vi "ScanEngine_SLM.vi"(7 "Action":T2, 8 "Metric Control":T3, 11 "Holo Array In":T1[](array[typedef]) {"Modes"."Amplititute" step=0.05}) -> (0 "Metric Image":sgl[][](array[numeric]), 2 "Metric Result":dbl)   [LabVIEW 2014]
uses:
  Controls/MetricControl_SLM.ctl
  Controls/Scan Metric_SLM.ctl
  Controls/ScanEngineState_SLM.ctl
  Controls/Holo Settings.ctl
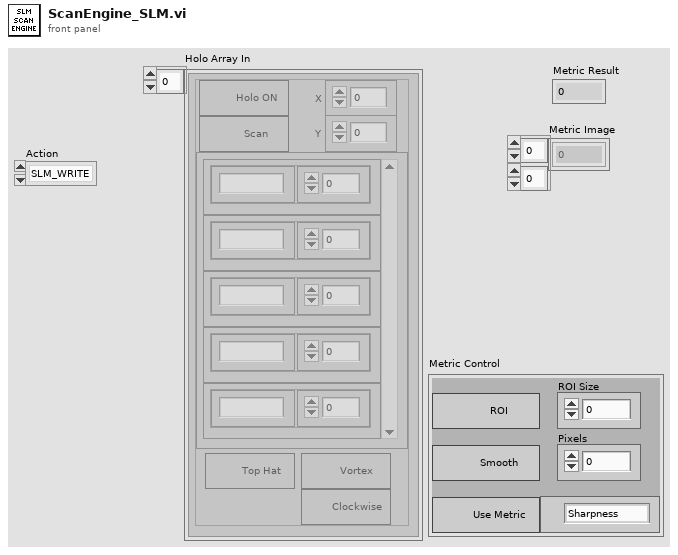
[diagram p1: front panel]
types:
  T1 = typedef "Holo Settings.ctl" = cluster{"Top Hat":bool, "Modes":cluster{"Mode ID":string, "Amplititute":dbl}[], "Vortex":bool, "Clockwise":bool, "X":dbl, "Y":dbl, "Holo ON":bool, "Scan":bool}
  T2 = typedef "ScanEngineState_SLM.ctl" = enum16{"SLM_WRITE", "IMAGE", ""}
  T3 = typedef "MetricControl_SLM.ctl" = cluster{"Use Metric":bool, "SLM Metric":T4, "Smooth":bool, "Pixels":dbl, "ROI":bool, "ROI Size":dbl}
  T4 = typedef "Scan Metric_SLM.ctl" = enum16{"Sharpness", "Brightness", "Combined"}
  T5 = typedef "Image Acquisition Parameters.ctl" = cluster{"Scan Type":enum16{"Sample Scanning", "Beam Scanning"}, "Scan Mode":enum16{"XY", "XZ", "YZ", "XYZ"}, "Fast Axis Frequency (Hz)":dbl, "Image Format":u16, "Line Accumulations":u16, "Frames Per Capture":u16, "Frames Accumulations":u16, "Image Dimension (um)":dbl[], "Number of Z Steps":u8, "Z Steps Size (um)":dbl, "Pixel Size (nm)":dbl[]}
  T6 = typedef "SLM General Settings.ctl" = cluster{"Holo size (pixels)":i32, "Top hat radius":dbl, "Number of modes":i32, "Bkg gradient X":dbl, "Bkg gradient Y":dbl, "Flat":bool, "Mode Matrix":u16}
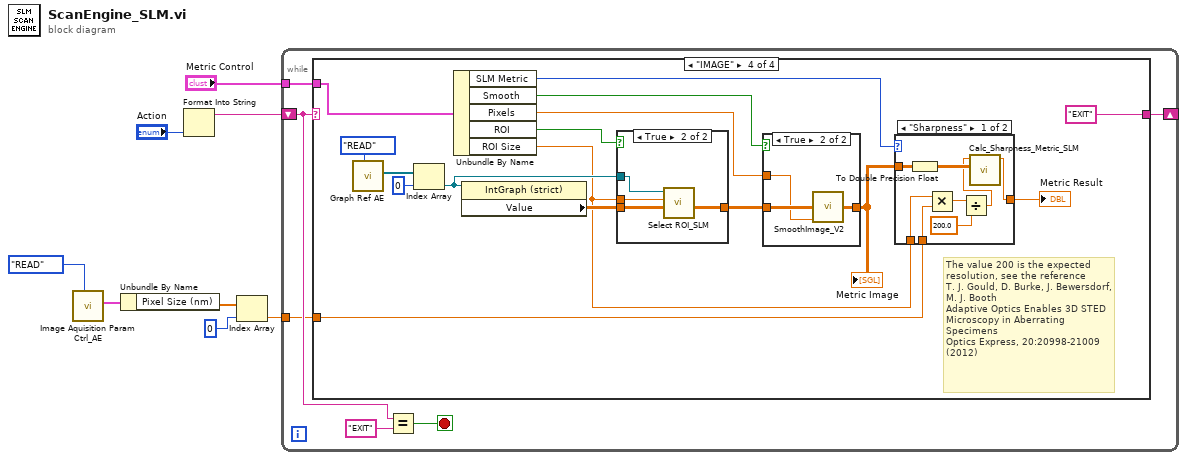
[diagram p0: block diagram]
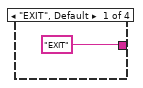
[diagram p2: hidden frame]
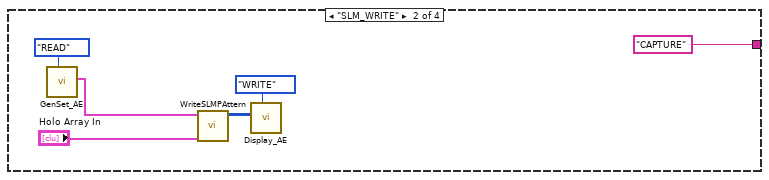
[diagram p3: hidden frame]
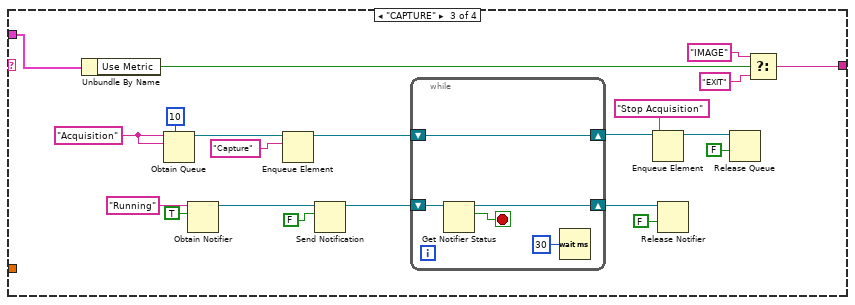
[diagram p4: hidden frame]
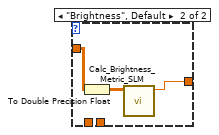
[diagram p6: hidden frame]
diagram:
  n1 = call "Image Aquisition Param Ctrl_AE.vi"("Action"=enum16{"READ", "WRITE"}."READ") -> ("Image Acquisition Parameters Out"=w4:T5)  [unwired: 10 in]
  n2 = Unbundle By Name(w4) -> ("Pixel Size (nm)"=w3:dbl[])
  n3 = Format Into String("Action") -> (resulting string=w6:string)  [unwired: 3 in, 1 out]
  n4 = Index Array(array=w3, index=0) -> (element=w1:dbl)
  n5 = while {
    shift-right: [w14] -> _
    shift-left: w6 -> [w13]
    tunnel: "Metric Control" -> [w10]
    tunnel: w1 -> [w9]
    stop <- w11 stop-if-true
    n6 = case shown="\"IMAGE\"" w13 {
      tunnel: ["EXIT" "CAPTURE" w39 "EXIT"] -> w14
      tunnel: w10 -> [_ _ w28 w60]
      tunnel: w9 -> [_ _ _ w48]
      frame "EXIT", Default {
      }
      frame "SLM_WRITE" {
        n7 = call "GenSet_AE.vi"("Enum"=enum16{"READ", "WRITE"}."READ") -> ("General settings Out"=w18:T6)  [unwired: 10 in]
        n8 = call "WriteSLMPAttern.vi"("Holo Array"="Holo Array In", "General settings"=w18) -> ("Display Array"=w17:u8[][])  [unwired: 9 in]
        n9 = call "Display_AE.vi"("Action"=enum16{"READ", "WRITE"}."WRITE", "Display Array In"=w17) -> ()  [unwired: 9 in, 1 out]
      }
      frame "CAPTURE" {
        w36 = "Acquisition" ("name (unnamed)")
        n10 = Unbundle By Name(w28) -> ("Use Metric"=w27:bool)
        n11 = Obtain Queue(max queue size (-1, unlimited)=10, name (unnamed)=w36, element data type=w36) -> (queue out=w34:refnum<queue>)  [unwired: 2 in, 2 out]
        n12 = Obtain Notifier(name (unnamed)="Running", notification data type=TRUE) -> (notifier out=w31:refnum<notifier>)  [unwired: 2 in, 2 out]
        n13 = Enqueue Element(queue=w34, element="Capture") -> (queue out=w24:refnum<queue>)  [unwired: 2 in, 2 out]
        n14 = Send Notification(notification=FALSE, notifier=w31) -> (notifier out=w40:refnum<notifier>)  [unwired: 1 in, 1 out]
        n15 = while {
          shift-right: [w43] -> w25
          shift-left: w24 -> [w43]
          shift-right: [w44] -> w30
          shift-left: w40 -> [w47]
          stop <- w46 stop-if-true
          n16 = Get Notifier Status(notifier=w47) -> (notifier out=w44:refnum<notifier>, current notification=w46:bool)  [unwired: 1 in, 3 out]
          n17 = Wait (ms)(milliseconds to wait=u32 30) -> ()  [unwired: 1 out]
        }
        n18 = Enqueue Element(queue=w25, element="Stop Acquisition") -> (queue out=w23:refnum<queue>)  [unwired: 2 in, 2 out]
        n19 = Release Notifier(notifier=w30, force destroy? (F)=FALSE) -> ()  [unwired: 1 in, 3 out]
        n20 = Release Queue(queue=w23, force destroy? (F)=FALSE) -> ()  [unwired: 1 in, 3 out]
        n21 = Select(t="IMAGE", s=w27, f="EXIT") -> (s? t:f=w39:string)
      }
      frame "IMAGE" {
        # "The value 200 is the expected\nresolution, see the reference\nT. J. Gould, D. Burke, J. Bewersdorf, M. J. Booth\nAdaptive Optics Enables 3D STED Microscopy in Aberrating Specimens\nOptics Express, 20:20998-21009 (2012)"
        n22 = call "Graph Ref AE.vi"("Action"=enum16{"READ", "WRITE"}."READ") -> ("Graph Ref Out"=w55:refnum<vi>[])  [unwired: 10 in]
        n23 = Index Array(array=w55, index=0) -> (element=w50:refnum<vi>)
        n24 = Unbundle By Name(w60) -> ("SLM Metric"=w59:T4, "Smooth"=w57:bool, "Pixels"=w58:dbl, "ROI"=w53:bool, "ROI Size"=w49:dbl)
        n25 = property class="IntGraph (strict)"(reference=w50) -> ("Value"=w51:sgl[][])  [unwired: 1 in, 2 out]
        n26 = case shown="True" w53 {
          tunnel: w51 -> [w64 w68]
          tunnel: [w64 w67] -> w52
          tunnel: w49 -> [_ w66]
          tunnel: w50 -> [_ w65]
          frame False {
          }
          frame True {
            n27 = call "Select ROI_SLM.vi"("Array In"=w68, "ROI Size"=w66, "IntensityGraph in"=w65) -> ("ROI"=w67:sgl[][])  [unwired: 8 in]
          }
        }
        n28 = case shown="True" w57 {
          tunnel: w52 -> [w80 w83]
          tunnel: [w80 w82] -> w63
          tunnel: w58 -> [_ w81]
          frame False {
          }
          frame True {
            n29 = call "SmoothImage_V2.vi"("Image IN"=w83, "Sigma (Radius)"=w81) -> ("Smoothed Image"=w82:sgl[][])  [unwired: 13 in]
          }
        }
        "Metric Image" <- w63
        n30 = case shown="\"Sharpness\"" w59 {
          tunnel: w63 -> [w76 w79]
          tunnel: [w74 w78] -> w61
          tunnel: w49 -> [w73 _]
          tunnel: w48 -> [w72 _]
          frame "Sharpness" {
            n31 = To Double Precision Float(number=w76) -> (double precision float=w75:dbl[][])
            n32 = Multiply(x=w73, y=w72) -> (x*y=w71:dbl)
            n33 = Divide(x=w71, y=200.0) -> (x/y=w69:dbl)
            n34 = call "Calc_Sharpness_Metric_SLM.vi"("AC Image"=w75, "Numeric in"=w69) -> ("Numeric out"=w74:dbl)  [unwired: 9 in]
          }
          frame "Brightness", Default {
            n35 = To Double Precision Float(number=w79) -> (double precision float=w77:dbl[][])
            n36 = call "Calc_Brightness_Metric_SLM.vi"("Image In"=w77) -> ("Brightness"=w78:dbl)  [unwired: 10 in]
          }
        }
        "Metric Result" <- w61
      }
    }
    n37 = Equal?(x=w13, y="EXIT") -> (x = y?=w11:bool)
  }
